vi "ROI_Cut2_Pic.vi"(8 "error in":errorcluster, 10 "Name":string, 11 "Image Org In":T1) -> (0 "error out":errorcluster, 3 "CutPath":path[](array[path]))   [LabVIEW 2019]
uses:
  <vilib>/vision/Image Controls.llb/IMAQ Image.ctl
  Function/UpVision/Ctrl/UpColorImg.ctl
  Auto Inspection Tray Map Name.ctl
  983d85d7-d574-4517-a0dc-21b930af5ff7.vi
  <vilib>/JDP Science/JSONtext/JSON text to Variant.vi
  Global/Process Global.vi
  <vilib>/vision/NI_Vision_Development_Module.lvlib
panel:
  out "Image":T1(plugin-control)
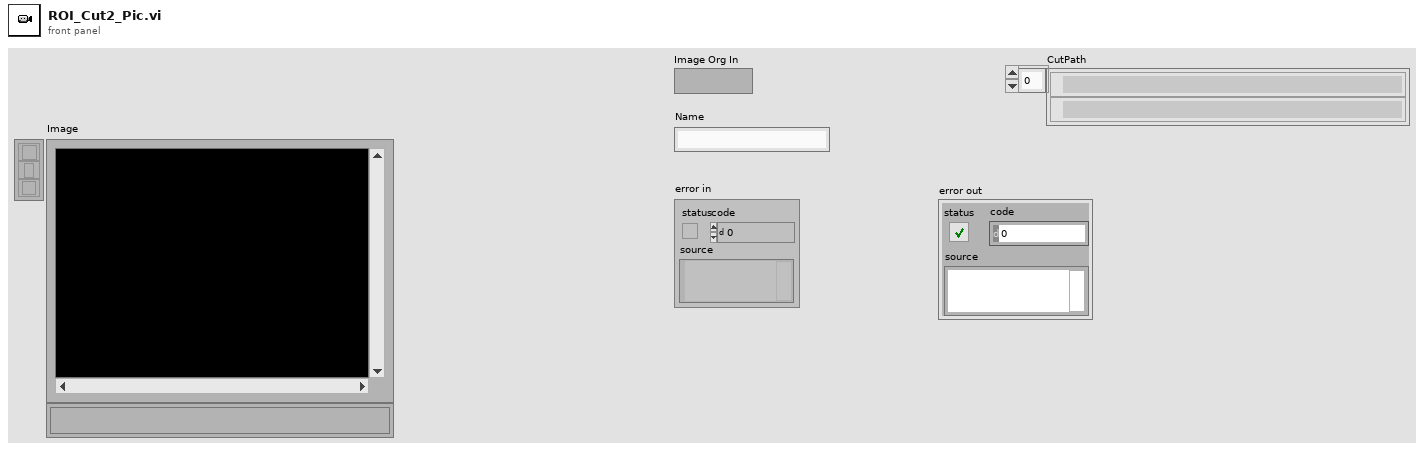
[diagram p1: front panel]
types:
  T1 = typedef "IMAQ Image.ctl" = refnum<image>
  T2 = typedef "Auto Inspection Tray Map Name.ctl" = enum16{"LSTable", "AITable", "LSMap", "AIMap"}
  T3 = typedef "UpColorImg.ctl" = enum16{"CUpCam", "CUpSource", "CUpShow", "CUpToProcess1", "CUpToProcess2", "CUpForMatch", "CUpForCheckNumbers", "CupPreProcess"}
  T4 = enum16{"Initial", "Write", "Read", "Save", "Load", "WrteAll"}
  T5 = cluster{"Global Rectangle":i32[], "Contours":cluster{"Contour Type":u32, "ROI Type":u32, "Points":i32[]}[]}
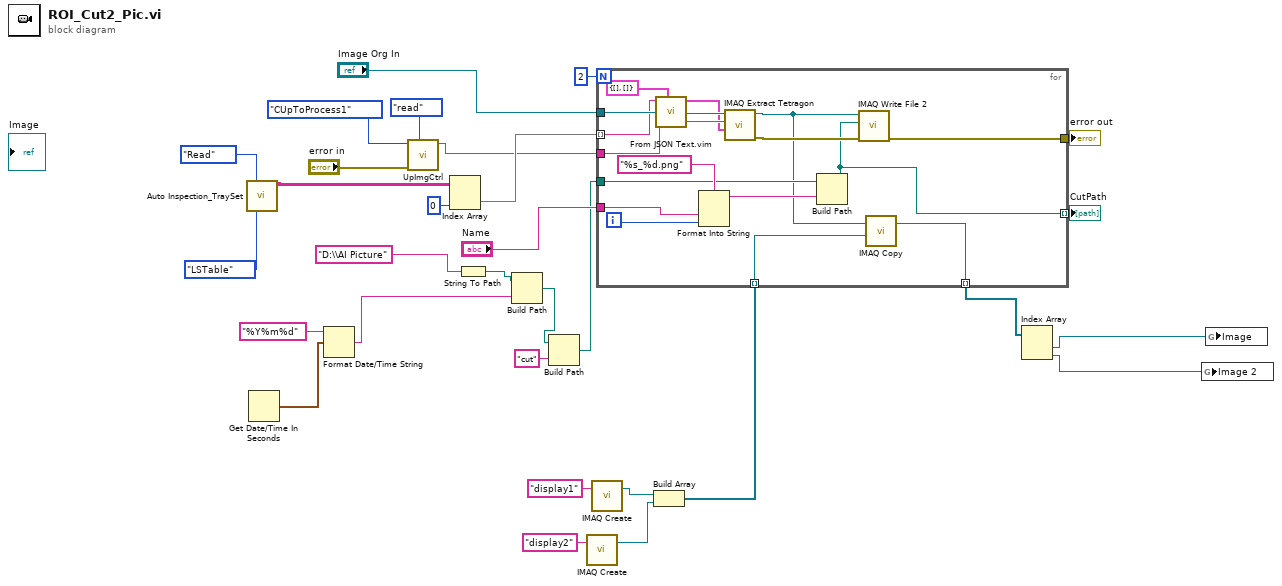
[diagram p0: block diagram]
diagram:
  n1 = call "Auto Inspection_TraySet.vi"("Action"=T4."Read", "Name"=Auto_Inspection_Tray_Map_Name."LSTable") -> ("LSTableOut"=w30:string[][])  [unwired: 8 in, 5 out]
  n2 = Get Date/Time In Seconds() -> (seconds since 1Jan1904=w8:timestamp)
  n3 = Format Date/Time String(time format string (%c)="%Y%m%d", seconds (now)=w8) -> (date/time string=w4:string)  [unwired: 1 out]
  n4 = call "UpImgCtrl.vi"("Action"=enum16{"Initial", "read", "release"}."read", "error in (no error)"="error in", "ColorImg 2"=UpColorImg."CUpToProcess1") -> ("ColorImg"=w22:string)  [unwired: 6 in, 2 out]
  n5 = Index Array(array=w30, index (col)=0 ("disabled index (col)")) -> (element=w29:string[])  [unwired: 1 in]
  n6 = String To Path(string="D:\\AI Picture") -> (path=w5:path)
  n7 = Build Path(base path=w5, name or relative path=w4) -> (appended path=w3:path)
  n8 = Build Path(base path=w3, name or relative path="cut") -> (appended path=w2:path)
  n9 = call "IMAQ Create"("Image Name"="display2") -> ("New Image"=w15:T1)  [unwired: 4 in, 1 out]
  n10 = call "IMAQ Create"("Image Name"="display1") -> ("New Image"=w16:T1)  [unwired: 4 in, 1 out]
  n11 = Build Array(w16, w15) -> (w14:T1[])
  n12 = for {
    N: 2 -> [_]
    tunnel: "Image Org In" -> [w46]
    tunnel: w22 -> [w45]
    tunnel: w29 -> [w44] mode=indexing
    tunnel: w2 -> [w35]
    tunnel: "Name" -> [w39]
    tunnel: [w36] -> w21
    tunnel: [w34] -> w18 mode=indexing
    tunnel: w14 -> [w33] mode=indexing
    tunnel: [w31] -> w13 mode=indexing
    i -> [w38]
    n13 = call "From JSON Text.vim"("Data Type and Default Value"=T5 {"Global Rectangle"=[], "Contours"=[]} ("ROI"), "JSON"=w44) -> ("Data out"=w42:T5)  [unwired: 8 in, 1 out]
    n14 = Format Into String(format string="%s_%d.png", w39, w38) -> (resulting string=w37:string)  [unwired: 2 in, 1 out]
    n15 = call-poly "IMAQ Extract Tetragon"("ROI Descriptor"=w42, "Image Dst"=w45, "Image Src"=w46) -> ("error out"=w41:errorcluster, "Image Dst Out"=w32:T1)  [unwired: 7 in]
    n16 = Build Path(base path=w35, name or relative path=w37) -> (appended path=w34:path)
    n17 = call-poly "IMAQ Write File 2"("error in (no error)"=w41, "File Path"=w34, "Image"=w32) -> ("error out"=w36:errorcluster)  [unwired: 7 in, 1 out]
    n18 = call "IMAQ Copy"("Image Dst"=w33, "Image Src"=w32) -> ("Image Dst Out"=w31:T1)  [unwired: 4 in, 1 out]
  }
  "error out" <- w21
  "CutPath" <- w18
  n19 = Index Array(array=w13) -> (element #1=w12:T1, element #2=w11:T1)  [unwired: 2 in]
  n20 = global write "Process Global.vi" "Image 2"(w11) -> ()
  n21 = global write "Process Global.vi" "Image"(w12) -> ()
